vi "ColorToRGB.vi"(0 "RED INPUT":dynamicdata(waveform), 1 "RED MIN":dbl, 2 "RED MAX":dbl, 3 "GREEN MIN":dbl, 4 "GREEN MAX":dbl, 6 "BLUE INPUT":dynamicdata(waveform), 7 "BLUE MIN":dbl, 8 "GREEN Sensitivity":dbl(slide)=1.0 scale=0.0..2.0, 9 "BLUE MAX":dbl, 10 "CLEAR INPUT":dynamicdata(waveform), 11 "RED Sensitivity":dbl(slide)=1.0 scale=0.0..2.0, 12 "GREEN INPUT":dynamicdata(waveform), 13 "BLUE Sensitivity":dbl(slide)=1.0 scale=0.0..2.0) -> (14 "G":dbl=-10.799485158466023 format="%#_3g", 15 "SENSOR OUTPUT":u32(colorbox), 16 "B":dbl=-9.75398695854645 format="%#_3g", 17 "Color Chart":T1(graph)={"Scalar"=148.2043560224322, "Scalar"=177.70606350859296, "Scalar"=472.56299264691984, "Scalar"=127.15641383309193}, 18 "R":dbl=-15.9759800739675 format="%#_3g")   [LabVIEW 2022 SP3]
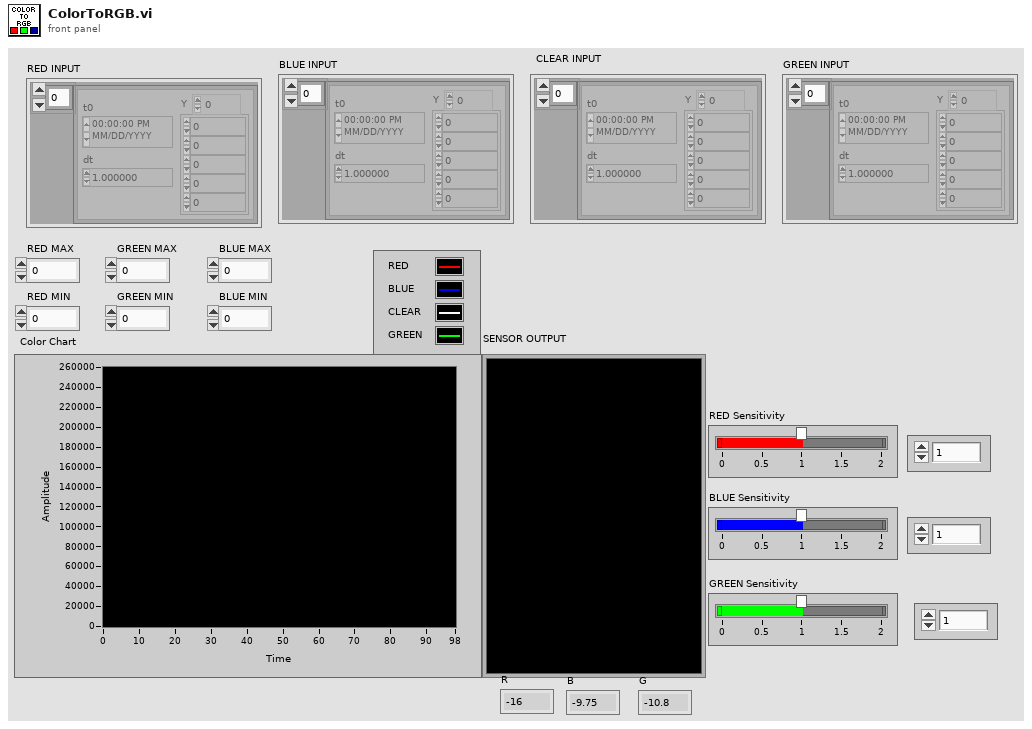
[diagram p1: front panel]
types:
  T1 = cluster{"Scalar":dbl, "Scalar":dbl, "Scalar":dbl, "Scalar":dbl}
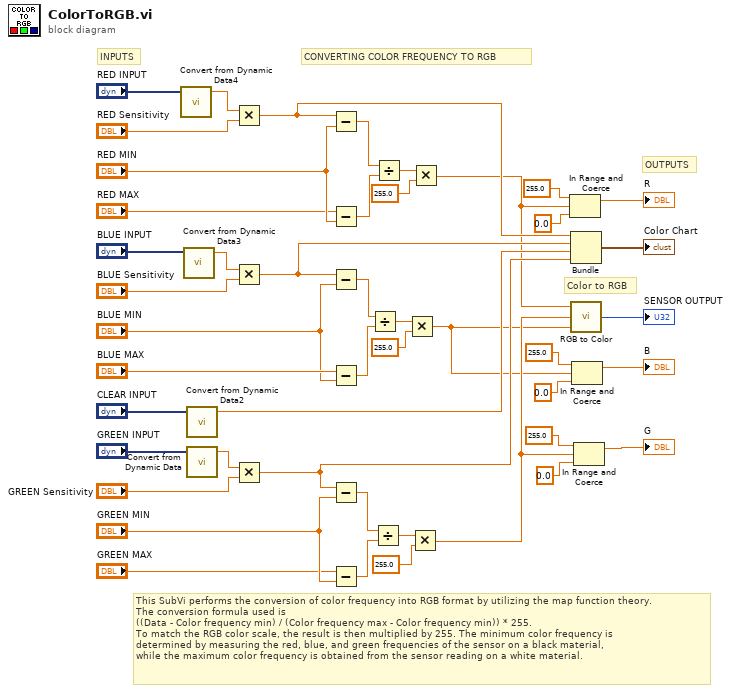
[diagram p0: block diagram]
diagram:
  # "This SubVi performs the conversion of color frequency into RGB format by utilizing the map function theory. \nThe conversion formula used is\n((Data - Color frequency min) / (Color frequency max - Color frequency min)) * 255. \nTo match the RGB color scale, the result is then multiplied by 255. The minimum color frequency is \ndetermined by measuring the red, blue, and green frequencies of the sensor on a black material, \nwhile the maximum color frequency is obtained from the sensor reading on a white material."
  # "Color to RGB"
  # "OUTPUTS"
  # "INPUTS"
  # "CONVERTING COLOR FREQUENCY TO RGB"
  n1 = call "Convert from Dynamic Data4"("Dynamic Data Type"="RED INPUT") -> ("Scalar"=w33:dbl)  [unwired: 3 in]
  n2 = call "Convert from Dynamic Data3"("Dynamic Data Type"="BLUE INPUT") -> ("Scalar"=w35:dbl)  [unwired: 3 in]
  n3 = call "Convert from Dynamic Data2"("Dynamic Data Type"="CLEAR INPUT") -> ("Scalar"=w20:dbl)  [unwired: 3 in]
  n4 = call "Convert from Dynamic Data"("Dynamic Data Type"="GREEN INPUT") -> ("Scalar"=w37:dbl)  [unwired: 3 in]
  n5 = Multiply(x=w33, y="RED Sensitivity") -> (x*y=w34:dbl)
  n6 = Multiply(x=w35, y="BLUE Sensitivity") -> (x*y=w36:dbl)
  n7 = Multiply(x=w37, y="GREEN Sensitivity") -> (x*y=w38:dbl)
  n8 = Subtract(x=w34, y="RED MIN") -> (x-y=w25:dbl)
  n9 = Subtract(x="RED MAX", y="RED MIN") -> (x-y=w24:dbl)
  n10 = Subtract(x=w36, y="BLUE MIN") -> (x-y=w29:dbl)
  n11 = Subtract(x="BLUE MAX", y="BLUE MIN") -> (x-y=w28:dbl)
  n12 = Subtract(x=w38, y="GREEN MIN") -> (x-y=w22:dbl)
  n13 = Subtract(x="GREEN MAX", y="GREEN MIN") -> (x-y=w21:dbl)
  n14 = Divide(x=w29, y=w28) -> (x/y=w27:dbl)
  n15 = Divide(x=w22, y=w21) -> (x/y=w31:dbl)
  n16 = Divide(x=w25, y=w24) -> (x/y=w23:dbl)
  n17 = Multiply(x=w27, y=255.0) -> (x*y=w2:dbl)
  n18 = Multiply(x=w31, y=255.0) -> (x*y=w12:dbl)
  n19 = Multiply(x=w23, y=255.0) -> (x*y=w6:dbl)
  n20 = In Range and Coerce(upper limit=255.0, x=w6, lower limit=0.0) -> (coerced(x)=→"R":dbl)  [unwired: 1 out]
  n21 = Bundle(w34, w36, "Scalar"=w20, w38) -> (→"Color Chart":cluster{dbl, dbl, "Scalar":dbl, dbl})  [unwired: 1 in]
  n22 = call <vilib>:"RGB to Color.vi"("B"=w2, "G"=w12, "R"=w6) -> ("Color"=→"SENSOR OUTPUT":u32)
  n23 = In Range and Coerce(upper limit=255.0, x=w2, lower limit=0.0) -> (coerced(x)=→"B":dbl)  [unwired: 1 out]
  n24 = In Range and Coerce(upper limit=255.0, x=w12, lower limit=0.0) -> (coerced(x)=→"G":dbl)  [unwired: 1 out]
